vi "Refresh.vi"(8 "error in (no error)":errorcluster, 10 "Force Refresh (F)":bool, 11 "Ethernet in":refnum<class "ENET_BS120x.lvclass">) -> (0 "error out":errorcluster, 3 "Ethernet out":refnum<class "ENET_BS120x.lvclass">)   [LabVIEW 2021, in "BS120x Driver.lvlib" / "ENET_BS120x.lvclass"]
doc: "Refreshes BS1200 UDP\nForce Refresh will guarantee a read timeout will occur. Default is true"
uses:
  ENET_BS120x.lvclass
  ENET_BS120x.lvclass/ENET_BS120x.ctl
  <vilib>/xnet/xnet.llb/XNET Frame CAN.ctl
  <vilib>/xnet/xnet.llb/XNET Frame Type CAN.ctl
  _Private/Data Classes/CAN Data Class/CAN Data.lvclass/CAN Data.ctl
  _Private/Data Classes/CAN Data Class/CAN Data.lvclass
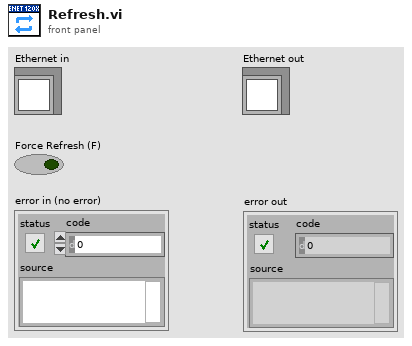
[diagram p1: front panel]
types:
  T1 = typedef "XNET Frame CAN.ctl" = cluster{"timestamp":timestamp, "payload":u8[], "identifier":u32, "type":T2, "extended?":bool, "echo?":bool}
  T2 = typedef "XNET Frame Type CAN.ctl" = u8
  T3 = cluster{"identifier":u32, "extended?":bool, "type":enum8{"CAN Data", "CAN Remote"}, "payload":u8[]}[]
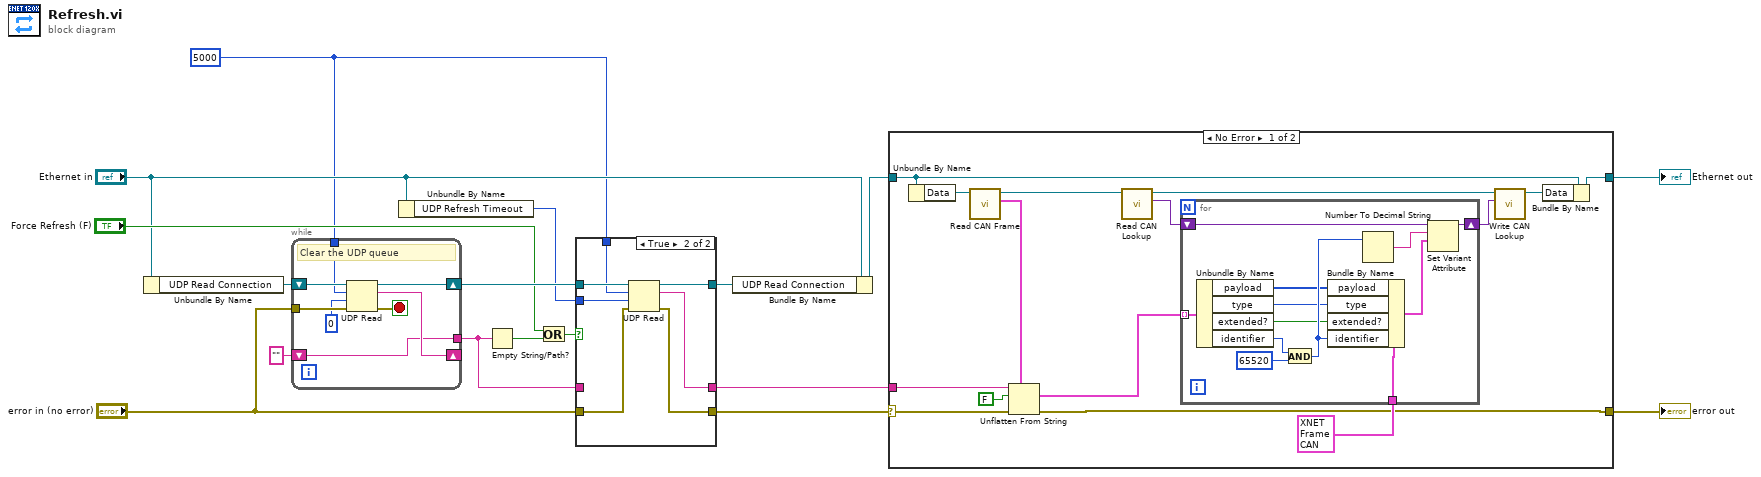
[diagram p0: block diagram]
diagram:
  w1 = 5000 ("max size (548)")
  n1 = Unbundle By Name("Ethernet in") -> ("UDP Read Connection"=w17:refnum<k16>)
  n2 = while {
    shift-right: [w23] -> w13
    shift-left: w17 -> [w24]
    shift-right: [w22] -> _
    shift-left: "" ("data out") -> [w19]
    tunnel: [w19] -> w14
    tunnel: "error in (no error)" -> [w25]
    tunnel: w1 -> [w18]
    stop <- w20 stop-if-true
    # "Clear the UDP queue"
    n3 = UDP Read(connection ID=w24, max size (548)=w18, timeout ms (25000)=0, 8:w25) -> (data out=w22:string, error out=w20:errorcluster, 3:w23:refnum<k16>)  [unwired: 2 out]
  }
  n4 = Unbundle By Name("Ethernet in") -> ("UDP Refresh Timeout"=w2:u16)
  n5 = Empty String/Path?(string/path=w14) -> (empty?=w11:bool)
  n6 = Or(x="Force Refresh (F)", y=w11) -> (x .or. y?=w8:bool)
  n7 = case shown="True" w8 {
    tunnel: [w28 w35] -> w7
    tunnel: w14 -> [w28 _]
    tunnel: [w27 w34] -> w6
    tunnel: "error in (no error)" -> [w27 w33]
    tunnel: w13 -> [w26 w32]
    tunnel: [w26 w31] -> w4
    tunnel: w2 -> [_ w30]
    tunnel: w1 -> [_ w29]
    frame False {
    }
    frame True {
      n8 = UDP Read(connection ID=w32, max size (548)=w29, timeout ms (25000)=w30, 8:w33) -> (data out=w35:string, error out=w34:errorcluster, 3:w31:refnum<k16>)  [unwired: 2 out]
    }
  }
  n9 = Bundle By Name(cluster="Ethernet in", "UDP Read Connection"=w4) -> (w5:refnum<class "ENET_BS120x.lvclass">)
  n10 = case shown="No Error" w6 {
    selector: w6 -> [w48 w63]
    tunnel: [w50 w64] -> w16
    tunnel: [w36 w63] -> w15
    tunnel: w7 -> [w49 _]
    tunnel: w5 -> [w47 w64]
    frame No Error {
      n11 = Unbundle By Name(w47) -> ("Data"=w46:refnum<class "CAN Data.lvclass">)
      n12 = call "Read CAN Frame.vi"("CAN Data in"=w46) -> ("CAN Frame Array"=w42:T3, "CAN Data out"=w44:refnum<class "CAN Data.lvclass">)  [unwired: 8 in, 1 out]
      n13 = Unflatten From String(type=w42, binary string=w49, data includes array or string size? (T)=FALSE, error in (no error)=w48) -> (value=w43:T3, error out=w36:errorcluster)  [unwired: 2 out]
      n14 = call "Read CAN Lookup.vi"("CAN Data in"=w44) -> ("CAN Lookup"=w39:variant, "CAN Data out"=w40:refnum<class "CAN Data.lvclass">)  [unwired: 8 in, 1 out]
      n15 = for {
        tunnel: w43 -> [w60] mode=indexing
        shift-right: [w58] -> w38
        shift-left: w39 -> [w59]
        tunnel: T1 {"timestamp"=timestamp(0 s since 1904-01-01), "payload"=[], "identifier"=0, "type"=0, "extended?"=FALSE, "echo?"=FALSE} ("CAN frame") -> [w54]
        n16 = Unbundle By Name(w60) -> ("payload"=w53:u8[], "type"=w52:enum8{"CAN Data", "CAN Remote"}, "extended?"=w51:bool, "identifier"=w61:u32)
        n17 = And(x=w61, y=u32 65520) -> (x .and. y?=w56:u32)
        n18 = Bundle By Name(cluster=w54, "payload"=w53, "type"=w52, "extended?"=w51, "identifier"=w56) -> (w57:T1)
        n19 = Number To Decimal String(number=w56) -> (decimal integer string=w55:string)  [unwired: 1 in]
        n20 = Set Variant Attribute(Variant=w59, name=w55, value=w57) -> (Variant out=w58:variant)  [unwired: 1 in, 2 out]
      }
      n21 = call "Write CAN Lookup.vi"("CAN Lookup"=w38, "CAN Data in"=w40) -> ("CAN Data out"=w41:refnum<class "CAN Data.lvclass">)  [unwired: 8 in, 1 out]
      n22 = Bundle By Name(cluster=w47, "Data"=w41) -> (w50:refnum<class "ENET_BS120x.lvclass">)
    }
    frame Error {
    }
  }
  "Ethernet out" <- w16
  "error out" <- w15
